vi "Analyse.vi"(8 "error in (no error)":errorcluster, 11 "IResultHandler in":refnum<class "IResultHandler.lvclass">) -> (0 "error out":errorcluster, 1 "ICallResult":refnum<class "ICallResult.lvclass">, 2 "Request ID":u64, 3 "IResultHandler out":refnum<class "IResultHandler.lvclass">)   [LabVIEW 2020, in "wamplv.lvlib" / "IResultHandler.lvclass"]
uses:
  IResultHandler.lvclass
  Call/ICallResult/ICallResult.lvclass
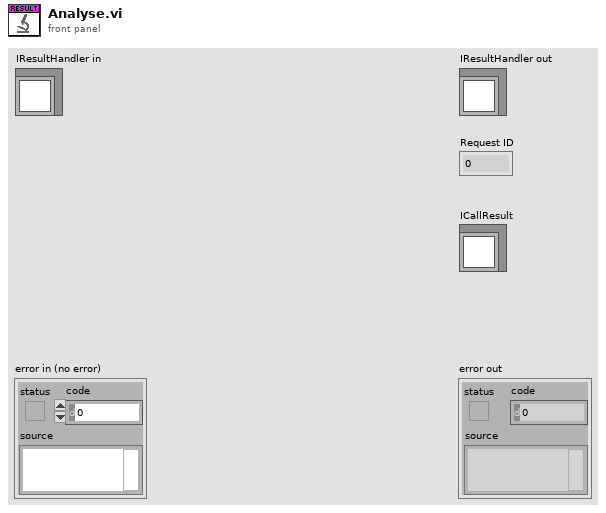
[diagram p1: front panel]
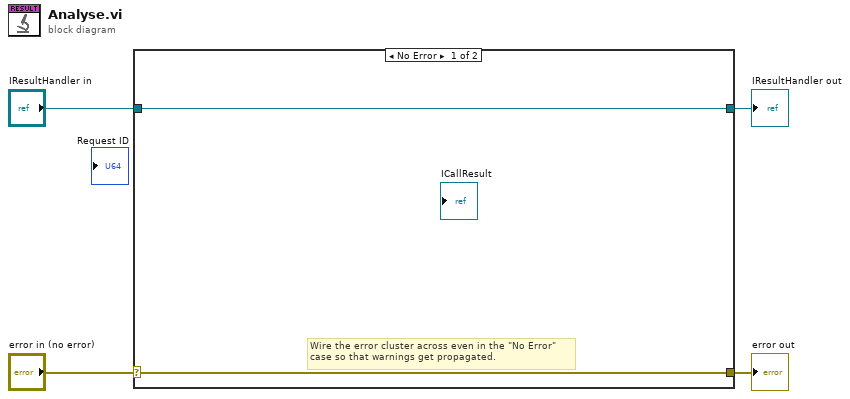
[diagram p0: block diagram]
diagram:
  n1 = case shown="No Error" "error in (no error)" {
    selector: "error in (no error)" -> [w5 w8]
    tunnel: [w5 w8] -> w3
    tunnel: [w6 w7] -> w1
    tunnel: "IResultHandler in" -> [w6 w7]
    frame No Error {
      # "Wire the error cluster across even in the \"No Error\"\ncase so that warnings get propagated."
    }
    frame Error {
    }
  }
  "error out" <- w3
  "IResultHandler out" <- w1
